vi "Task7.vi"() -> ()   [LabVIEW 2017]
panel:
  in  "Numeric 2":dbl
  out "Numeric":u16
  in  "Array":bool[](array[boolean])
  in  "0 - binary, 1 - octal, 2 - decimal, 3 - hexadecimal":u8(knob) scale=0.0..3.0
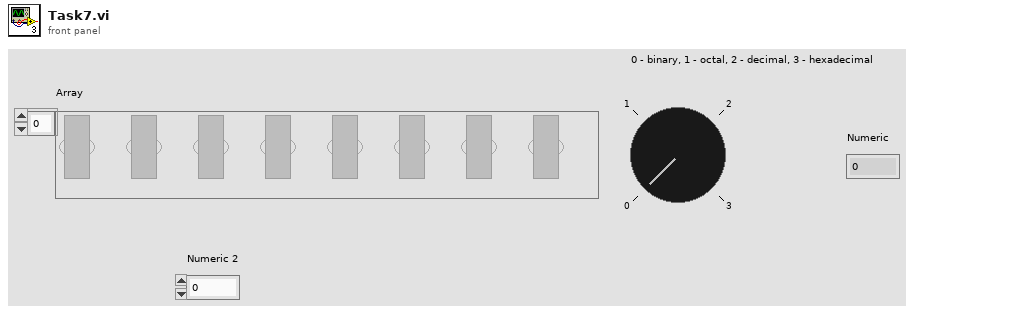
[diagram p1: front panel]
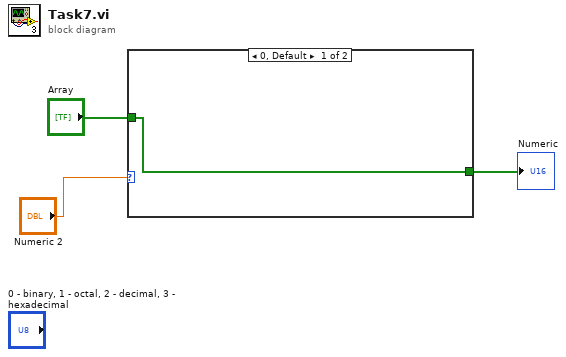
[diagram p0: block diagram]
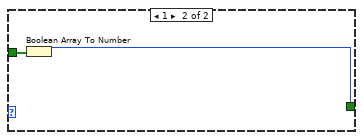
[diagram p2: hidden frame]
diagram:
  n1 = case shown="0, Default" "Numeric 2" {
    tunnel: "Array" -> [w4 w6]
    tunnel: [w4 w5] -> w2
    frame 0, Default {
    }
    frame 1 {
      n2 = Boolean Array To Number(Boolean array=w6) -> (number=w5:u32)
    }
  }
  "Numeric" <- w2
